vi "EventReason_SM.vi"(8 "error in (no error)":errorcluster, 10 "EventReason":string, 11 "Inspection Statemachine in":refnum<class "Inspection Statemachine.lvclass">) -> (0 "error out":errorcluster, 3 "Inspection Statemachine out":refnum<class "Inspection Statemachine.lvclass">)   [LabVIEW 2019, in "Inspection Statemachine.lvclass"]
uses:
  Inspection Statemachine.lvclass
  <vilib>/event_ctls.llb/usereventprio.ctl
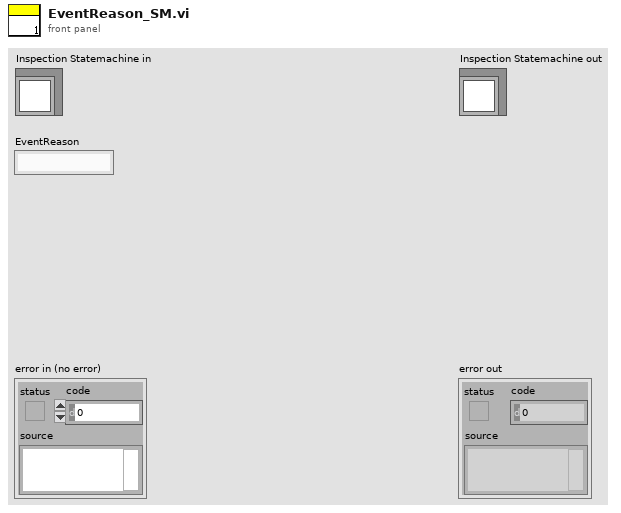
[diagram p1: front panel]
types:
  T1 = typedef "usereventprio.ctl" = enum32{"high priority", "normal priority"}
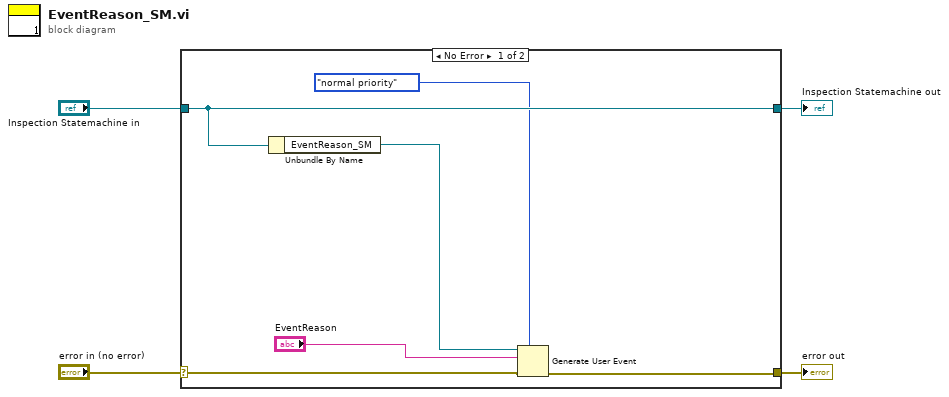
[diagram p0: block diagram]
diagram:
  n1 = case shown="No Error" "error in (no error)" {
    selector: "error in (no error)" -> [w9 w12]
    tunnel: [w8 w12] -> w3
    tunnel: [w10 w11] -> w1
    tunnel: "Inspection Statemachine in" -> [w10 w11]
    frame No Error {
      n2 = Unbundle By Name(w10) -> ("EventReason_SM"=w7:refnum<user-event>)
      n3 = Generate User Event(priority (normal)=usereventprio."normal priority", user event=w7, event data cluster="EventReason", error in=w9) -> (error out=w8:errorcluster)  [unwired: 1 out]
    }
    frame Error {
    }
  }
  "error out" <- w3
  "Inspection Statemachine out" <- w1
